vi "5.7.5-Midbrain-How-UDPClient.vi"() -> ()   [LabVIEW 2010]
doc: "This VI implements a client for the Named Service UDP Server.vi.\nIt connects to a service by specifying the server address and the name of the service. After sending a 'Hello' string to the server, the client receives the string sent by the server, displays the string and closes the connection.\n\n<b>Note:</b> This VI is built to work with the Named Service UDP Server.vi in UDP.llb."
uses:
  4-High Neurons/4.4-How Sensor Typedef.ctl
  4-High Neurons/4.0-Midbrain State.ctl
  5.0-Global.vi
panel:
  out "5.4.4 How Am I? Sensor":T1
  out "address":u32
  out "port":u16
  out "String":string
  out "Error Out":errorcluster
  in  "Error In":errorcluster
  # "Instructions:\n1. Open Named Service UDP Server.vi located in the same library.\n2. Follow the instructions on it's front panel.\n\nNote: This VI is built to work with the Named Service UDP Server.vi in UDP.llb."
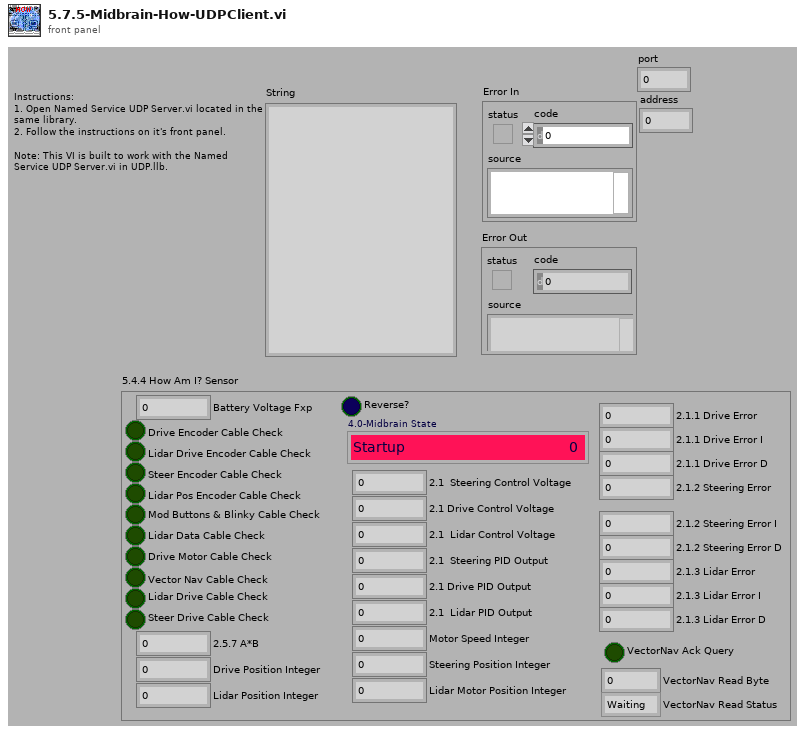
[diagram p1: front panel]
types:
  T1 = typedef "4.4-How Sensor Typedef.ctl" = cluster{"Motor Speed Integer":i32, "Drive Position Integer":i32, "Lidar Position Integer":i32, "Lidar Motor Position Integer":i32, "Steering Position Integer":i32, "Battery Voltage Fxp":dbl, "Drive Encoder Cable Check":bool, "Lidar Drive Encoder Cable Check":bool, "Steer Encoder Cable Check":bool, "Lidar Pos Encoder Cable Check":bool, "Mod Buttons & Blinky Cable Check":bool, "Lidar Data Cable Check":bool, "Drive Motor Cable Check":bool, "Vector Nav Cable Check":bool, "Lidar Drive Cable Check":bool, "Steer Drive Cable Check":bool, "Reverse?":bool, "2.1  Steering Control Voltage":dbl, "2.1 Drive Control Voltage":dbl, "2.1  Lidar Control Voltage":dbl, "2.5.7 A*B":dbl, "2.1  Steering PID Output":dbl, "2.1 Drive PID Output":dbl, "2.1  Lidar PID Output":dbl, "2.1.1 Drive Error":dbl, "2.1.1 Drive Error I":dbl, "2.1.1 Drive Error D":dbl, "2.1.2 Steering Error":dbl, "2.1.2 Steering Error I":dbl, "2.1.2 Steering Error D":dbl, "2.1.3 Lidar Error":dbl, "2.1.3 Lidar Error I":dbl, "2.1.3 Lidar Error D":dbl, "VectorNav Ack Query":bool, "VectorNav Read Byte":u8, "VectorNav Read Status":enum16{"Waiting", "Reading", "Done"}, "4.0-Midbrain State":T2}
  T2 = typedef "4.0-Midbrain State.ctl" = enum16{"Startup", "Waiting to Run", "Running-OlinOval", "Running-ChannelFollow", "Running-WallFollow", "Running-OpenTransit", "Running-Joystick Training", "Shutdown", "Restart", "New IP"}
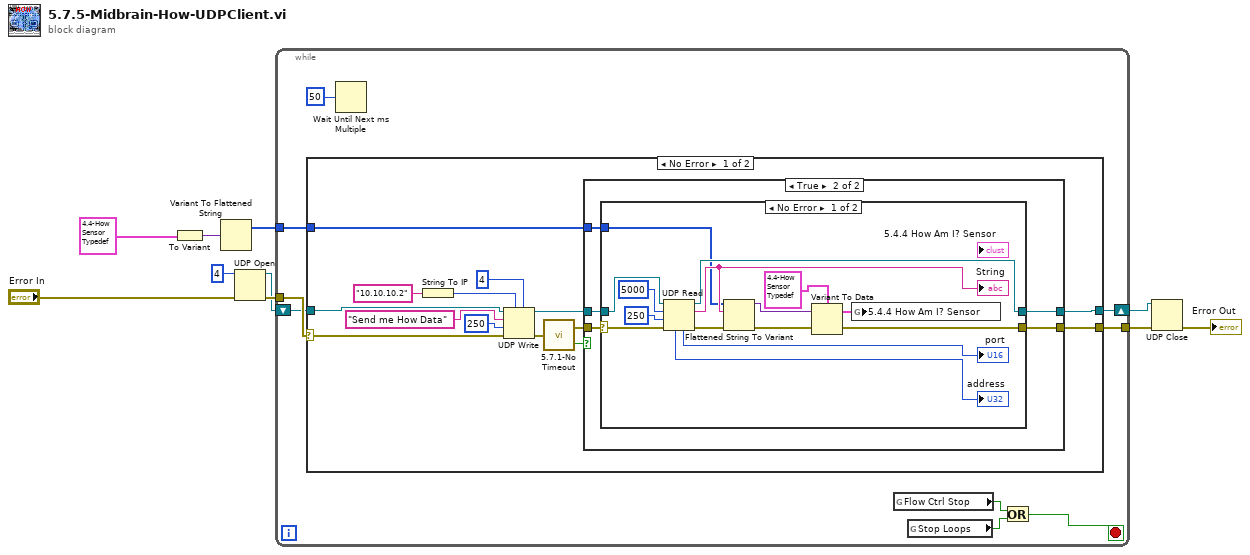
[diagram p0: block diagram]
diagram:
  n1 = To Variant(anything=T1 {"Motor Speed Integer"=0, "Drive Position Integer"=0, "Lidar Position Integer"=0, "Lidar Motor Position Integer"=0, "Steering Position Integer"=0, "Battery Voltage Fxp"=0.0, "Drive Encoder Cable Check"=FALSE, "Lidar Drive Encoder Cable Check"=FALSE, "Steer Encoder Cable Check"=FALSE, "Lidar Pos Encoder Cable Check"=FALSE, "Mod Buttons & Blinky Cable Check"=FALSE, "Lidar Data Cable Check"=FALSE, "Drive Motor Cable Check"=FALSE, "Vector Nav Cable Check"=FALSE, "Lidar Drive Cable Check"=FALSE, "Steer Drive Cable Check"=FALSE, "Reverse?"=FALSE, "2.1  Steering Control Voltage"=0.0, "2.1 Drive Control Voltage"=0.0, "2.1  Lidar Control Voltage"=0.0, "2.5.7 A*B"=0.0, "2.1  Steering PID Output"=0.0, "2.1 Drive PID Output"=0.0, "2.1  Lidar PID Output"=0.0, "2.1.1 Drive Error"=0.0, "2.1.1 Drive Error I"=0.0, "2.1.1 Drive Error D"=0.0, "2.1.2 Steering Error"=0.0, "2.1.2 Steering Error I"=0.0, "2.1.2 Steering Error D"=0.0, "2.1.3 Lidar Error"=0.0, "2.1.3 Lidar Error I"=0.0, "2.1.3 Lidar Error D"=0.0, "VectorNav Ack Query"=FALSE, "VectorNav Read Byte"=0, "VectorNav Read Status"=enum."Waiting", "4.0-Midbrain State"=enum."Startup"} ("5.4.4 How Am I? Sensor")) -> (Variant=w3:variant)
  n2 = Variant To Flattened String(Variant=w3) -> (1:w4:i16[])  [unwired: 1 out]
  n3 = UDP Open(8:"Error In", 11:u16 4 ("port")) -> (port=w8:refnum<k16>, 0:w9:errorcluster)  [unwired: 3 in, 1 out]
  n4 = while {
    tunnel: [w19] -> w6
    tunnel: w9 -> [w18]
    shift-right: [w16] -> w7
    shift-left: w8 -> [w17]
    tunnel: w4 -> [w15]
    stop <- w11 stop-if-true
    n5 = case shown="No Error" w18 {
      selector: w18 -> [w33 w59]
      tunnel: [w28 w59] -> w19
      tunnel: w17 -> [w32 w58]
      tunnel: [w27 w58] -> w16
      tunnel: w15 -> [w22 _]
      frame No Error {
        n6 = String To IP(1:"10.10.10.2" ("Forbrain IP")) -> (0:w31:u32)
        n7 = UDP Write(address=w31, port or service name=u16 4, connection ID=w32, data in="Send me How Data", 8:w33, 9:250 ("timeout ms (25000)")) -> (error out=w26:errorcluster, 3:w29:refnum<k16>)
        n8 = call "5.7.1-No Timeout.vi"("error in (no error)"=w26) -> ("No Timeout"=w24:bool, "error out"=w25:errorcluster)
        n9 = case shown="True" w24 {
          tunnel: w25 -> [w35 w40]
          tunnel: w29 -> [w34 w39]
          tunnel: [w34 w38] -> w27
          tunnel: [w35 w37] -> w28
          tunnel: w22 -> [_ w36]
          frame False {
          }
          frame True {
            n10 = case shown="No Error" w40 {
              selector: w40 -> [w55 w56]
              tunnel: w39 -> [w54 w57]
              tunnel: [w52 w57] -> w38
              tunnel: [w45 w56] -> w37
              tunnel: w36 -> [w49 _]
              frame No Error {
                n11 = UDP Read(connection ID=w54, max size (548)=5000, timeout ms (25000)=250, 8:w55) -> (data out=w50:string, error out=w46:errorcluster, 3:w52:refnum<k16>, 4:→"port":u16, 6:→"address":u32)
                "String" <- w50
                n12 = Flattened String To Variant(4:w46, 6:w50, 7:w49) -> (0:w47:errorcluster, 3:w48:variant)
                n13 = Variant To Data(error in=w47, Variant=w48, type=T1 {"Motor Speed Integer"=0, "Drive Position Integer"=0, "Lidar Position Integer"=0, "Lidar Motor Position Integer"=0, "Steering Position Integer"=0, "Battery Voltage Fxp"=0.0, "Drive Encoder Cable Check"=FALSE, "Lidar Drive Encoder Cable Check"=FALSE, "Steer Encoder Cable Check"=FALSE, "Lidar Pos Encoder Cable Check"=FALSE, "Mod Buttons & Blinky Cable Check"=FALSE, "Lidar Data Cable Check"=FALSE, "Drive Motor Cable Check"=FALSE, "Vector Nav Cable Check"=FALSE, "Lidar Drive Cable Check"=FALSE, "Steer Drive Cable Check"=FALSE, "Reverse?"=FALSE, "2.1  Steering Control Voltage"=0.0, "2.1 Drive Control Voltage"=0.0, "2.1  Lidar Control Voltage"=0.0, "2.5.7 A*B"=0.0, "2.1  Steering PID Output"=0.0, "2.1 Drive PID Output"=0.0, "2.1  Lidar PID Output"=0.0, "2.1.1 Drive Error"=0.0, "2.1.1 Drive Error I"=0.0, "2.1.1 Drive Error D"=0.0, "2.1.2 Steering Error"=0.0, "2.1.2 Steering Error I"=0.0, "2.1.2 Steering Error D"=0.0, "2.1.3 Lidar Error"=0.0, "2.1.3 Lidar Error I"=0.0, "2.1.3 Lidar Error D"=0.0, "VectorNav Ack Query"=FALSE, "VectorNav Read Byte"=0, "VectorNav Read Status"=enum."Waiting", "4.0-Midbrain State"=enum."Startup"} ("5.4.4 How Am I? Sensor")) -> (error out=w45:errorcluster, data=w41:T1)
                n14 = global write "5.0-Global.vi" "5.4.4 How Am I? Sensor"(w41) -> ()
              }
              frame Error {
              }
            }
          }
        }
      }
      frame Error {
      }
    }
    n15 = Wait Until Next ms Multiple(millisecond multiple=u32 50) -> ()  [unwired: 1 out]
    n16 = global read "5.0-Global.vi" "Flow Ctrl Stop"() -> (w13:bool)
    n17 = global read "5.0-Global.vi" "Stop Loops"() -> (w12:bool)
    n18 = Or(x=w13, y=w12) -> (x .or. y?=w11:bool)
  }
  n19 = UDP Close(connection ID=w7, 8:w6) -> (error out=→"Error Out":errorcluster)  [unwired: 1 out]
